vi "On Click New Config.vi"(8 "error in (no error)":errorcluster, 11 "App in":refnum<class "App.lvclass">) -> (0 "error out":errorcluster, 3 "App out":refnum<class "App.lvclass">)   [LabVIEW 2020, in "AR Example.lvlib" / "App.lvclass"]
uses:
  App.lvclass
  UI/Tab Control.ctl
  g_ar_toolkit.capture/Stream/Camera Parameter Information.ctl
  App.lvclass/App.ctl
  UI/UI.lvclass
  g_ar_toolkit.capture/Stream/Stream.lvclass
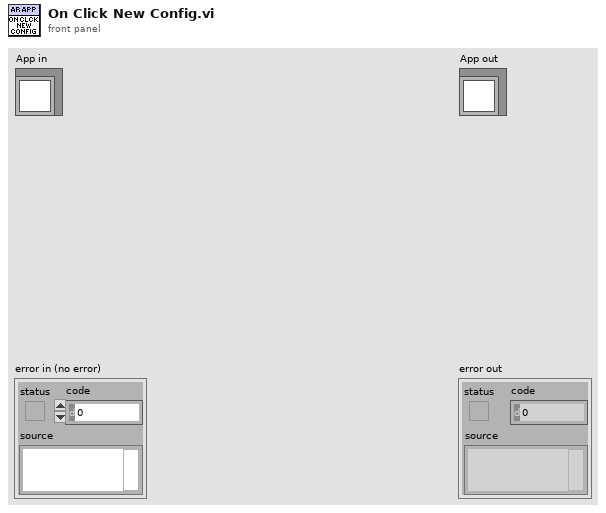
[diagram p1: front panel]
types:
  T1 = typedef "g_ar_toolkit.capture.lvlib/Stream.lvclass/Camera Parameter Information.ctl" = cluster{"Is Supported":bool, "Max":i32, "Min":i32, "Step":i32, "Default":i32}
  T2 = typedef "AR Example.lvlib/UI.lvclass/Tab Control.ctl" = enum8{"Config Load", "Camera Selection", "Camera Calibration"}
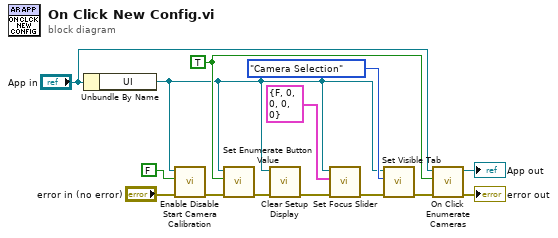
[diagram p0: block diagram]
diagram:
  w8 = TRUE ("Value")
  n1 = Unbundle By Name("App in") -> ("UI"=w2:refnum<class "UI.lvclass">)
  n2 = call-dynamic "Enable Disable Start Camera Calibration.vi"("error in (no error)"="error in (no error)", "Enable?"=FALSE, "UI in"=w2) -> ("error out"=w9:errorcluster)  [unwired: 8 in]
  n3 = call-dynamic "Set Enumerate Button Value.vi"("error in (no error)"=w9, "Values"=w8, "UI in"=w2) -> ("error out"=w10:errorcluster)  [unwired: 8 in]
  n4 = call-dynamic "Clear Setup Display.vi"("error in (no error)"=w10, "UI in"=w2) -> ("error out"=w6:errorcluster)  [unwired: 9 in]
  n5 = call "Set Focus Slider.vi"("error in (no error)"=w6, "Camera Parameter Information"=T1 {"Is Supported"=FALSE, "Max"=0, "Min"=0, "Step"=0, "Default"=0}, "UI in"=w2) -> ("error out"=w3:errorcluster)  [unwired: 8 in]
  n6 = call-dynamic "Set Visible Tab.vi"("error in (no error)"=w3, "Value"=Tab_Control."Camera Selection", "UI in"=w2) -> ("error out"=w5:errorcluster)  [unwired: 8 in]
  n7 = call "On Click Enumerate Cameras.vi"("error in (no error)"=w5, "Value"=w8, "App in"="App in") -> ("error out"=→"error out":errorcluster, "App out"=→"App out":refnum<class "App.lvclass">)  [unwired: 7 in]
